vi "Write NS Connection Msg.vi"(10 "GUI.lvlib:Network Stream.lvlib:NS Connection Msg.lvclass":refnum<class "NS Connection Msg.lvclass">, 11 "Network Stream in":refnum<class "Network Stream.lvclass">) -> (3 "Network Stream out":refnum<class "Network Stream.lvclass">)   [LabVIEW 2019, in "Network Stream.lvlib" / "Network Stream.lvclass"]
uses:
  Network Stream.lvclass
  Network Stream Messages/NS Connection Msg/NS Connection Msg.lvclass
  Network Stream.lvclass/Network Stream.ctl
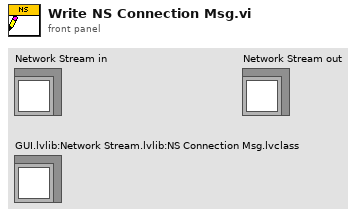
[diagram p1: front panel]
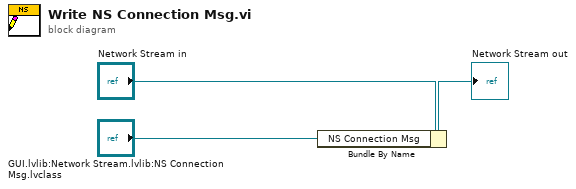
[diagram p0: block diagram]
diagram:
  n1 = Bundle By Name(cluster="Network Stream in", "NS Connection Msg"="GUI.lvlib:Network Stream.lvlib:NS Connection Msg.lvclass") -> (→"Network Stream out":refnum<class "Network Stream.lvclass">)
